vi "CRYSet Equation Front Panel.vi"(11 "Vi Ref":refnum<vi>) -> ()   [LabVIEW 2013]
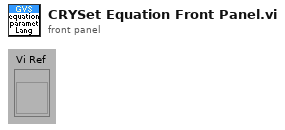
[diagram p1: front panel]
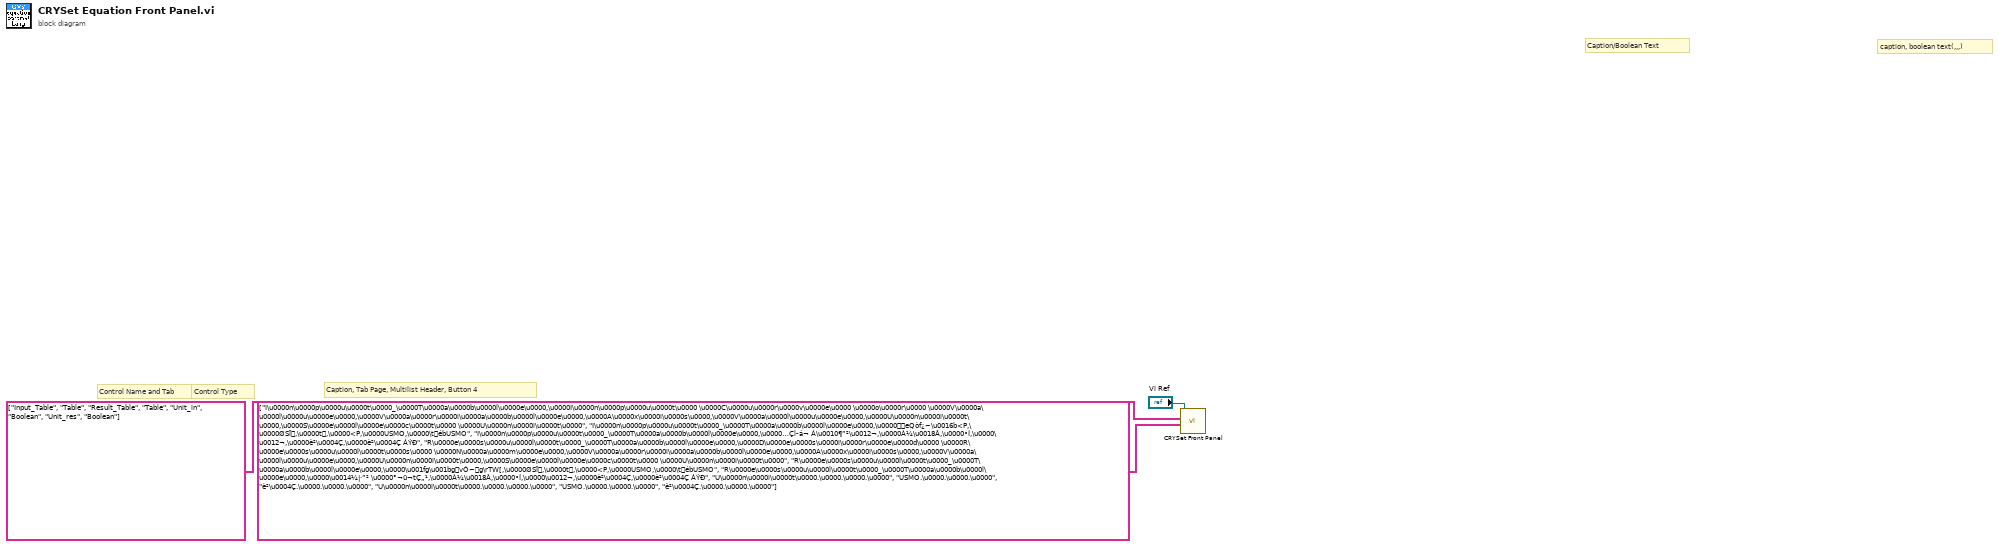
[diagram p0: block diagram]
diagram:
  # "Caption, Tab Page, Multilist Header, Button 4"
  # "Control Type"
  # "Control Name and Tab"
  # "caption, boolean text(,,,)"
  # "Caption/Boolean Text"
  n1 = call "CRYSet Front Panel.vi"("Caption(Boolean Text)"=string[][] [["I\u0000n\u0000p\u0000u\u0000t\u0000_\u0000T\u0000a\u0000b\u0000l\u0000e\u0000,\u0000I\u0000n\u0000p\u0000u\u0000t\u0000 \u0000C\u0000u\u0000r\u0000v\u0000e\u0000 \u0000o\u0000r\u0000 \u0000V\u0000a\u0000l\u0000u\u0000e\u0000,\u0000V\u0000a\u0000r\u0000i\u0000a\u0000b\u0000l\u0000e\u0000,\u0000A\u0000x\u0000i\u0000s\u0000,\u0000V\u0000a\u0000l\u0000u\u0000e\u0000,\u0000U\u0000n\u0000i\u0000t\u0000,\u0000S\u0000e\u0000l\u0000e\u0000c\u0000t\u0000 \u0000U\u0000n\u0000i\u0000t\u0000", "I\u0000n\u0000p\u0000u\u0000t\u0000_\u0000T\u0000a\u0000b\u0000l\u0000e\u0000,\u0000eQòf¿~\u0016b<P,\u0000ØSÏ,\u0000t,\u0000<P,\u0000USMO,\u0000\tébUSMO", "I\u0000n\u0000p\u0000u\u0000t\u0000_\u0000T\u0000a\u0000b\u0000l\u0000e\u0000,\u0000…Çl­á¬ Á\u0010¶”²\u0012¬,\u0000À¼\u0018Â,\u0000•Í,\u0000\u0012¬,\u0000è²\u0004Ç,\u0000è²\u0004Ç ÁÝÐ"], ["R\u0000e\u0000s\u0000u\u0000l\u0000t\u0000_\u0000T\u0000a\u0000b\u0000l\u0000e\u0000,\u0000D\u0000e\u0000s\u0000i\u0000r\u0000e\u0000d\u0000 \u0000R\u0000e\u0000s\u0000u\u0000l\u0000t\u0000s\u0000 \u0000N\u0000a\u0000m\u0000e\u0000,\u0000V\u0000a\u0000r\u0000i\u0000a\u0000b\u0000l\u0000e\u0000,\u0000A\u0000x\u0000i\u0000s\u0000,\u0000V\u0000a\u0000l\u0000u\u0000e\u0000,\u0000U\u0000n\u0000i\u0000t\u0000,\u0000S\u0000e\u0000l\u0000e\u0000c\u0000t\u0000 \u0000U\u0000n\u0000i\u0000t\u0000", "R\u0000e\u0000s\u0000u\u0000l\u0000t\u0000_\u0000T\u0000a\u0000b\u0000l\u0000e\u0000,\u0000\u001fg\u001bgvÓ~g\rTW[,\u0000ØSÏ,\u0000t,\u0000<P,\u0000USMO,\u0000\tébUSMO", "R\u0000e\u0000s\u0000u\u0000l\u0000t\u0000_\u0000T\u0000a\u0000b\u0000l\u0000e\u0000,\u0000\u0014¼|·”² \u0000°¬ü¬tÇ„¹,\u0000À¼\u0018Â,\u0000•Í,\u0000\u0012¬,\u0000è²\u0004Ç,\u0000è²\u0004Ç ÁÝÐ"], ["U\u0000n\u0000i\u0000t\u0000.\u0000.\u0000.\u0000", "USMO.\u0000.\u0000.\u0000", "è²\u0004Ç.\u0000.\u0000.\u0000"], ["U\u0000n\u0000i\u0000t\u0000.\u0000.\u0000.\u0000", "USMO.\u0000.\u0000.\u0000", "è²\u0004Ç.\u0000.\u0000.\u0000"]], "Control ID and Type(Label Name, Type)"=string[][] [["Input_Table", "Table"], ["Result_Table", "Table"], ["Unit_in", "Boolean"], ["Unit_res", "Boolean"]], "Vi Ref"="Vi Ref") -> ()  [unwired: 9 in]
